vi "004_FinalesCarrera_LDR_Zumbador.vi"() -> ()   [LabVIEW 2019]
uses:
  <vilib>/MakerHub/LINX/Public/Peripherals/Analog/Analog Read N Chans.vi
  <vilib>/MakerHub/LINX/Public/Peripherals/Analog/Analog Read 1 Chan.vi
  <vilib>/MakerHub/LINX/Public/Peripherals/Digital/Digital Write 1 Chan.vi
  <vilib>/MakerHub/LINX/Private/Local IO/LinxAnalogRead.vi
  <vilib>/MakerHub/LINX/Public/Utilities/Check Channel.vi
  <vilib>/MakerHub/LINX/Public/Peripherals/Digital/Digital Write N Chans.vi
  <vilib>/MakerHub/LINX/Private/Local IO/LinxDigitalWrite.vi
  <vilib>/MakerHub/LINX/Public/Utilities/Open Serial.vi
  <vilib>/MakerHub/LINX/Public/Sensors/Motion/Servo/Servo Open One Channel.vi
  <vilib>/MakerHub/LINX/Public/Sensors/Motion/Servo/Servo Set Pulse Width One Channel.vi
  <vilib>/MakerHub/LINX/Private/Utilties/Generate Error.vi
  <vilib>/MakerHub/LINX/Public/Sensors/Motion/Servo/Servo Close One Channel.vi
  <vilib>/MakerHub/LINX/LMH-LINX.lvlib
  <vilib>/MakerHub/LINX/Public/Sensors/Motion/Servo/Servo.lvlib
panel:
  out "VOLTAJE LDR":dbl
  in  "Zumbador":bool
  out "?":bool[](array[boolean])
  out "Voltages":dbl[](array[numeric])
  in  "Servo Position 2":u16(knob)=1493 scale=500.0..2500.0
  in  "Stop Button 2":bool
  in  "Serial Port 2":refnum<visa-resource-name>
  # "Servo Position \n(Pulse Width uS)"
  # "LINX Device Settings"
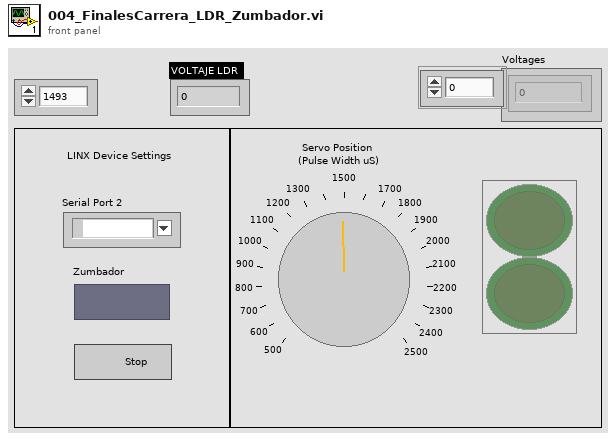
[diagram p1: front panel]
types:
  T1 = typedef "LMH-LINX.lvlib/LINX Ref.ctl" = cluster{"IO":T2, "Interface":T3, "LINX Device Config":T4}
  T2 = typedef "LMH-LINX.lvlib/Platform.ctl" = enum16{"Remote", "Local"}
  T3 = typedef "LMH-LINX.lvlib/Interface.ctl" = enum16{"Serial", "TCP"}
  T4 = typedef "LMH-LINX.lvlib/Device.lvlib/LINX Device Config.ctl" = cluster{"Interface":T3, "COM Port":refnum<visa-resource-name>, "TCP Configuration":T5, "Device Family":u8, "Device ID":u8, "Device Name":string, "TCP Ref":refnum<k5>, "Channels":T6}
  T5 = typedef "LMH-LINX.lvlib/Device.lvlib/TCP Config.ctl" = cluster{"IP Address":string, "Port":u16}
  T6 = typedef "LMH-LINX.lvlib/Channels.ctl" = cluster{"DI":u8[], "DO":u8[], "AI":u8[], "AO":u8[], "PWM":u8[], "QE":u8[], "UART":u8[], "I2C 2":u8[], "SPI":u8[], "CAN":u8[], "Servo":u8[], "AI Ref (V)":dbl, "AI Resolution (Bits)":u8, "AO Ref (V)":dbl, "AO Resolution (Bits)":u8}
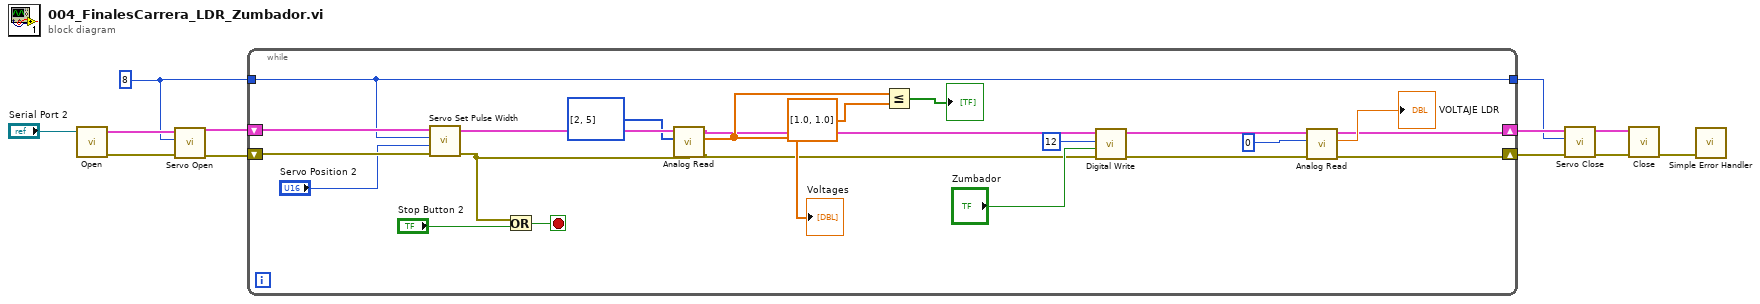
[diagram p0: block diagram]
diagram:
  w1 = u8 8 ("Servo Channel")
  n1 = call-poly <vilib>:"Open.vi"("Serial Port"="Serial Port 2") -> ("Error Out"=w12:errorcluster, "LINX Resource"=w11:T1)  [unwired: 8 in, 1 out]
  n2 = call-poly <vilib>:"Servo Open.vi"("Error In"=w12, "Servo Channel"=w1, "LINX Resource"=w11) -> ("Error Out"=w10:errorcluster, "LINX Resource"=w9:T1)  [unwired: 7 in]
  n3 = while {
    shift-right: [w13] -> w4
    shift-left: w10 -> [w29]
    tunnel: w1 -> [w27]
    shift-right: [w14] -> w7
    shift-left: w9 -> [w28]
    tunnel: [w27] -> w3
    stop <- w30 stop-if-true
    n4 = call-poly <vilib>:"Servo Set Pulse Width.vi"("Error In"=w29, "Pulse Width (uS)"="Servo Position 2", "Servo Channel"=w27, "LINX Resource"=w28) -> ("Error Out"=w23:errorcluster, "LINX Resource"=w24:T1)  [unwired: 6 in]
    n5 = Or(x=w23, y="Stop Button 2") -> (x .or. y?=w30:bool)
    n6 = call-poly <vilib>:"Analog Read.vi"("Error In"=w23, "AI Channel(s)"=u8[] [2, 5] ("AO Channel(s)"), "LINX Resource"=w24) -> ("Error Out"=w13:errorcluster, "Voltages"=w21:dbl[], "LINX Resource"=w14:T1)  [unwired: 5 in, 1 out]
    "Voltages" <- w21
    n7 = Less Or Equal?(x=w21, y=dbl[] [1.0, 1.0]) -> (x <= y?=→"?":bool[])
    n8 = call-poly <vilib>:"Digital Write.vi"("Error In"=w13, "Output Value"="Zumbador", "DO Channel"=u8 12, "LINX Resource"=w14) -> ()  [unwired: 6 in, 2 out]
    n9 = call-poly <vilib>:"Analog Read.vi"("Error In"=w13, "Analog Channel"=u8 0, "LINX Resource"=w14) -> ("Voltage"=→"VOLTAJE LDR":dbl)  [unwired: 5 in, 3 out]
  }
  n10 = call-poly <vilib>:"Servo Close.vi"("Error In"=w4, "Servo Channel"=w3, "LINX Resource"=w7) -> ("Error Out"=w5:errorcluster, "LINX Resource"=w6:T1)  [unwired: 7 in]
  n11 = call <vilib>:"Close.vi"("Error In"=w5, "LINX Resource"=w6) -> ("Error Out"=w8:errorcluster)  [unwired: 9 in]
  n12 = call <vilib>:"Simple Error Handler.vi"("error in (no error)"=w8) -> ()  [unwired: 4 in, 5 out]
